vi "RMS error (percent).vi"(2 "Target data":sgl[](array[numeric]) format="%.2f", 3 "ANN outputs":sgl[](array[numeric]) format="%.2f") -> (0 "%RMS":sgl format="%.2f")   [LabVIEW 2010]
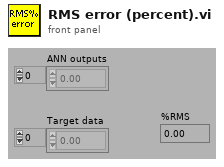
[diagram p1: front panel]
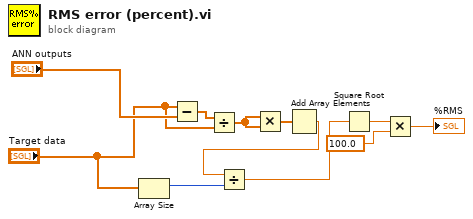
[diagram p0: block diagram]
diagram:
  n1 = Array Size(array="Target data") -> (size(s)=w1:i32)
  n2 = Subtract(x="Target data", y="ANN outputs") -> (x-y=w5:sgl[])
  n3 = Divide(x=w5, y="Target data") -> (x/y=w8:sgl[])
  n4 = Multiply(x=w8, y=w8) -> (x*y=w6:sgl[])
  n5 = Add Array Elements(numeric array=w6) -> (sum=w3:sgl)
  n6 = Divide(x=w3, y=w1) -> (x/y=w2:sgl)
  n7 = Square Root(x=w2) -> (sqrt(x)=w9:sgl)
  n8 = Multiply(x=w9, y=sgl 100.0) -> (x*y=→"%RMS":sgl)
